vi "Print Console.vi"() -> ()   [LabVIEW 2010]
doc: "This print queue console simulates the control of print job submissions and monitors the status of the print jobs being processed."
uses:
  Print LEDs.ctl
  Print Processing States.ctl
panel:
  out "Print LEDs":T1={"Waiting"=TRUE, "Initializing"=FALSE, "Printing"=FALSE}
  out "Queued Print Jobs":i32(slide) scale=0.0..25.0
  in  "Queue Event":bool
  in  "stop":bool
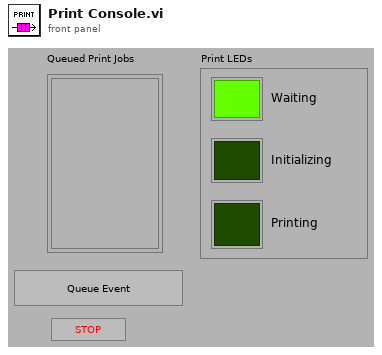
[diagram p1: front panel]
types:
  T1 = typedef "Print LEDs.ctl" = cluster{"Waiting":bool, "Initializing":bool, "Printing":bool}
  T2 = typedef "Print Processing States.ctl" = enum16{"Wait", "Initialize Setup", "Setup", "Initialize Print", "Print"}
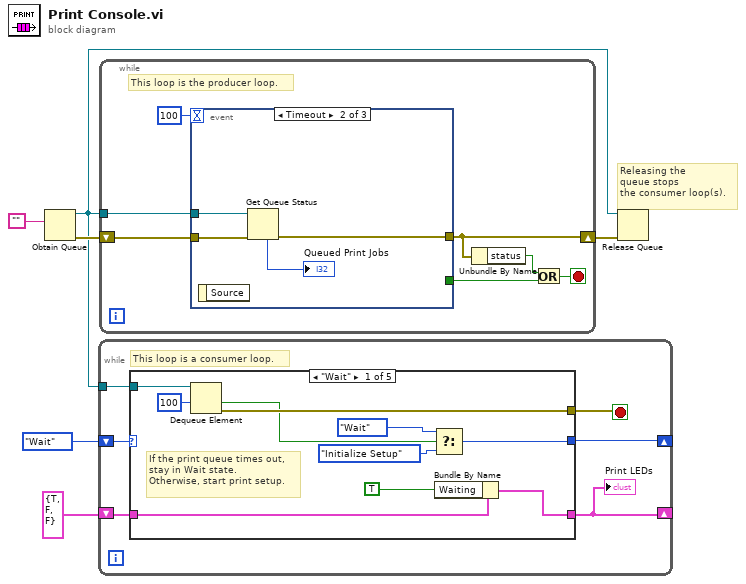
[diagram p0: block diagram]
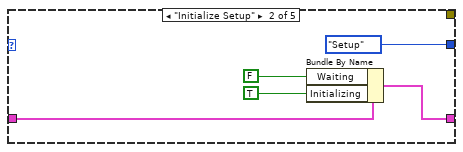
[diagram p2: hidden frame]
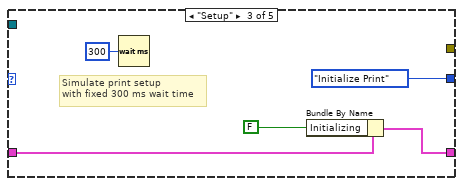
[diagram p3: hidden frame]
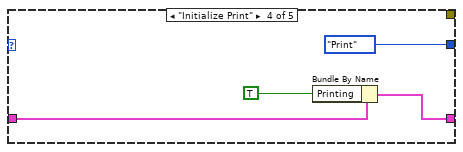
[diagram p4: hidden frame]
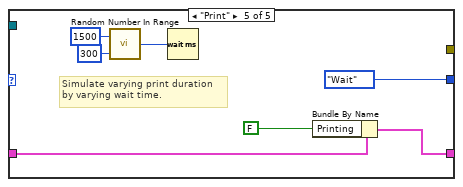
[diagram p5: hidden frame]
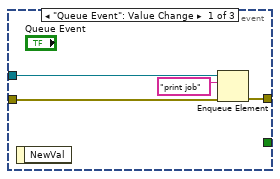
[diagram p6: hidden frame]
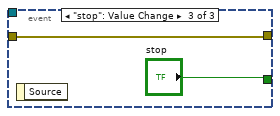
[diagram p7: hidden frame]
diagram:
  # "Releasing the\nqueue stops\nthe consumer loop(s)."
  n1 = Obtain Queue(element data type="") -> (queue out=w3:refnum<queue>, error out=w6:errorcluster)  [unwired: 4 in, 1 out]
  n2 = while {
    tunnel: w3 -> [w12]
    shift-right: [w9] -> _
    shift-left: Print_Processing_States."Wait" ("Enum") -> [w11]
    shift-right: [w7] -> _
    shift-left: T1 {"Waiting"=TRUE, "Initializing"=FALSE, "Printing"=FALSE} ("Print LEDs") -> [w10]
    stop <- w8 stop-if-true
    # "This loop is a consumer loop."
    n3 = case shown="\"Wait\"" w11 {
      tunnel: w12 -> [w22 _ _ _ _]
      tunnel: [w21 _ _ _ _] -> w8
      tunnel: w10 -> [w16 w26 w31 w35 w42]
      tunnel: [w15 w25 w30 w34 w41] -> w7
      tunnel: [w13 Print_Processing_States."Setup" ("Enum") Print_Processing_States."Initialize Print" ("Enum") Print_Processing_States."Print" ("Enum") Print_Processing_States."Wait" ("Enum")] -> w9
      frame "Wait" {
        # "If the print queue times out, \nstay in Wait state.\nOtherwise, start print setup."
        n4 = Dequeue Element(queue=w22, timeout in ms (-1)=100) -> (timed out?=w14:bool, error out=w21:errorcluster)  [unwired: 1 in, 2 out]
        n5 = Select(t=Print_Processing_States."Wait" ("Enum"), s=w14, f=Print_Processing_States."Initialize Setup" ("Enum")) -> (s? t:f=w13:T2)
        n6 = Bundle By Name(cluster=w16, "Waiting"=TRUE ("Waiting for\nnew job...")) -> (w15:T1)
      }
      frame "Initialize Setup" {
        n7 = Bundle By Name(cluster=w26, "Waiting"=FALSE ("Waiting for\nnew job..."), "Initializing"=TRUE ("Waiting for\nnew job...")) -> (w25:T1)
      }
      frame "Setup" {
        # "Simulate print setup\nwith fixed 300 ms wait time"
        n8 = Wait (ms)(milliseconds to wait=u32 300) -> ()  [unwired: 1 out]
        n9 = Bundle By Name(cluster=w31, "Initializing"=FALSE ("Waiting for\nnew job...")) -> (w30:T1)
      }
      frame "Initialize Print" {
        n10 = Bundle By Name(cluster=w35, "Printing"=TRUE ("Waiting for\nnew job...")) -> (w34:T1)
      }
      frame "Print" {
        # "Simulate varying print duration\nby varying wait time."
        n11 = call "Random Number In Range.vi"("Lower Limit"=u32 300, "Upper Limit"=u32 1500) -> ("Random #"=w37:u32)
        n12 = Wait (ms)(milliseconds to wait=w37) -> ()  [unwired: 1 out]
        n13 = Bundle By Name(cluster=w42, "Printing"=FALSE ("Waiting for\nnew job...")) -> (w41:T1)
      }
    }
    "Print LEDs" <- w7
  }
  n14 = while {
    shift-right: [w46] -> w5
    shift-left: w6 -> [w49]
    tunnel: w3 -> [w50]
    stop <- w47 stop-if-true
    # "This loop is the producer loop."
    n15 = event shown="[1] Timeout" {
      selector: _ -> [_ _ _]
      dyn-events: _ -> [_ _ _]
      timeout: 100 -> [_ _ _]
      tunnel: w50 -> [w54 w56 _]
      tunnel: w49 -> [w53 w57 w59]
      tunnel: [w52 w55 w59] -> w46
      tunnel: [_ _ "stop"] -> w48
      event "Queue Event": Value Change {
        n16 = event-data() -> ()  [unwired: 1 in, 1 out]
        n17 = Enqueue Element(queue=w54, element="print job", error in (no error)=w53) -> (error out=w52:errorcluster)  [unwired: 1 in, 2 out]
      }
      event Timeout {
        n18 = event-data() -> ()  [unwired: 1 in, 1 out]
        n19 = Get Queue Status(queue=w56, error in (no error)=w57) -> (error out=w55:errorcluster, # elements in queue=→"Queued Print Jobs":i32)  [unwired: 1 in, 6 out]
      }
      event "stop": Value Change {
        n20 = event-data() -> ()  [unwired: 1 in, 1 out]
      }
    }
    n21 = Unbundle By Name(w46) -> ("status"=w45:bool)
    n22 = Or(x=w45, y=w48) -> (x .or. y?=w47:bool)
  }
  n23 = Release Queue(queue=w3, error in (no error)=w5) -> ()  [unwired: 1 in, 3 out]
